vi "calculateAngle.vi"() -> ()   [LabVIEW 2018]
panel:
  out "End Angle":dbl(knob) scale=-180.0..180.0
  in  "Robot's Wanted Angle":i32
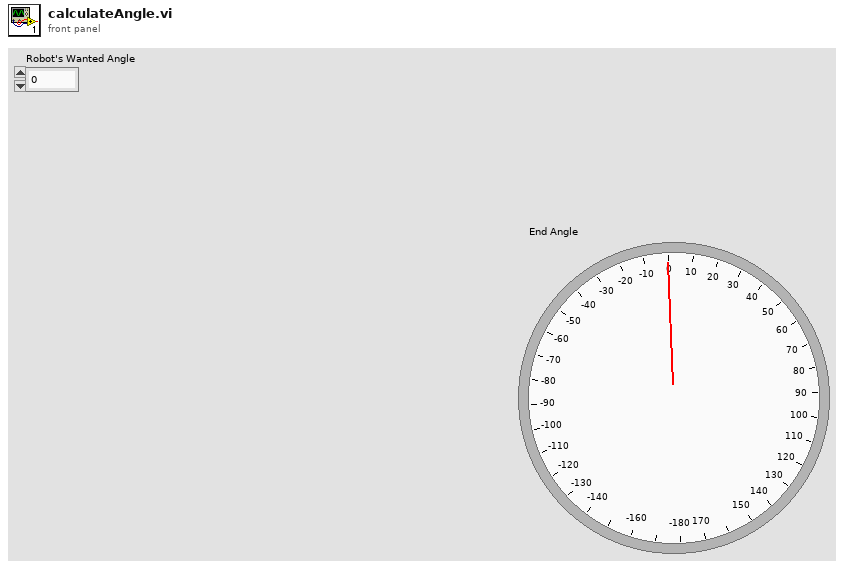
[diagram p1: front panel]
types:
  T1 = enum16{"[0, 360]", "[-180, 180]", "[0, 2PI]", "[-PI, PI]"}
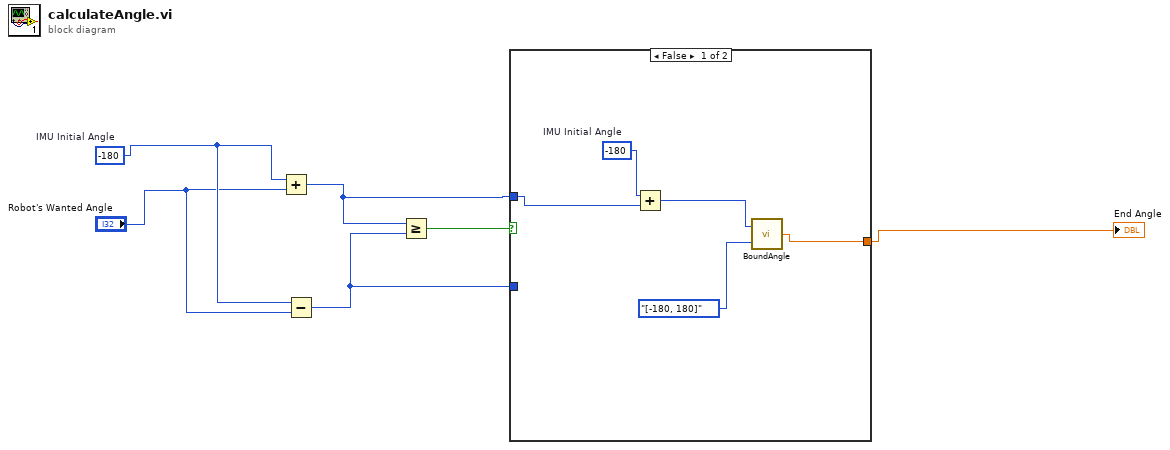
[diagram p0: block diagram]
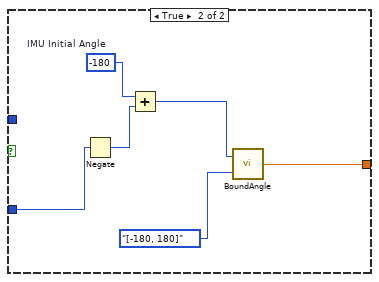
[diagram p2: hidden frame]
diagram:
  w6 = -180  # IMU Initial Angle
  n1 = Add(x=w6, y="Robot's Wanted Angle") -> (x+y=w2:i32)
  n2 = Subtract(x=w6, y="Robot's Wanted Angle") -> (x-y=w3:i32)
  n3 = Greater Or Equal?(x=w2, y=w3) -> (x >= y?=w4:bool)
  n4 = case shown="False" w4 {
    tunnel: w3 -> [_ w15]
    tunnel: [w7 w12] -> w1
    tunnel: w2 -> [w10 _]
    frame False {
      w9 = -180  # IMU Initial Angle
      n5 = Add(x=w9, y=w10) -> (x+y=w8:i32)
      n6 = call <userlib>:"BoundAngle.vi"("Type"=T1."[-180, 180]", "Angle"=w8) -> ("Bound Angle"=w7:dbl)
    }
    frame True {
      w16 = -180  # IMU Initial Angle
      n7 = Negate(x=w15) -> (-x=w14:i32)
      n8 = Add(x=w16, y=w14) -> (x+y=w13:i32)
      n9 = call <userlib>:"BoundAngle.vi"("Type"=T1."[-180, 180]", "Angle"=w13) -> ("Bound Angle"=w12:dbl)
    }
  }
  "End Angle" <- w1
